vi "FGV Numeric.vi"() -> (3 "Numeric UE":refnum<user-event>)   [LabVIEW 2024, in "User Events.lvlib"]
uses:
  User Events.lvlib
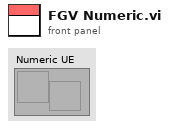
[diagram p1: front panel]
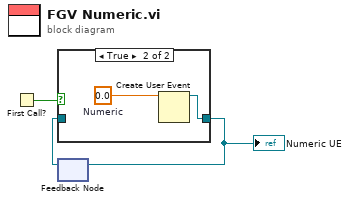
[diagram p0: block diagram]
diagram:
  n1 = First Call?() -> (First Call?: T/F=w1:bool)
  n2 = feedback #1() -> (w2:refnum<user-event>)  [unwired: 1 in]
  n3 = case shown="True" w1 {
    tunnel: [w4 w5] -> w3
    tunnel: w2 -> [w4 _]
    frame False {
    }
    frame True {
      w6 = 0.0  # Numeric
      n4 = Create User Event(user event datatype=w6) -> (user event=w5:refnum<user-event>)  [unwired: 1 in, 1 out]
    }
  }
  "Numeric UE" <- w3
  n5 = feedback-in #1(w3) -> ()
